vi "Configure Std Waveform.vi"(8 "error in":errorcluster, 11 "PXI-5441 Base CFG in":refnum<class "Fgen PXI CFG.lvclass">) -> (0 "error out":errorcluster, 3 "PXI-5441 Base CFG out":refnum<class "Fgen PXI CFG.lvclass">)   [LabVIEW 2023, in "HAL.lvlib" / "Fgen PXI.lvlib" / "Fgen PXI CFG.lvclass"]
uses:
  Fgen PXI CFG.lvclass
  Fgen PXI CFG.lvclass/Fgen PXI CFG.ctl
  fa98a2d5-c00a-4cbb-8575-3b170b0d9527.vi
  40d9fa99-6e9d-4d4b-a497-ff6c6c91f011.vi
  39bc53b2-902a-46e0-870e-d1b180cb98a6.vi
  c84aae48-2aac-49bb-a882-aaa71fe0ff4d.vi
  88318bc4-6f44-423c-ba11-5ee261214349.vi
  f3b2cb75-d808-412b-ab71-56c7bac84bdb.vi
  <vilib>/Utility/error.llb/Error Cluster From Error Code.vi
  <vilib>/ErrorRing/Error Ring.xnode
  4b2b93ff-10dc-4bd6-99e3-792703dd87f6.vi
  8e81885c-b6e8-4d7e-a9af-adfcbd4d7785.vi
  66779a04-485d-425c-828e-f39c11026279.vi
  Configuration Base/Configuration Base.lvclass
  fa7ec643-692d-4ae6-94d1-5cd9ea2710ab.vi
  <instrlib>/niFgen/niFgen.llb/niFgen Waveform Type.ctl
  <instrlib>/niFgen/niFgen.llb/niFgen Trigger Mode.ctl
  <instrlib>/niFgen/niFgen.llb/niFgen Output Mode.ctl
  D:/git/HAL/Configuration Base/Configuration Base.lvclass
  D:/git/HAL/Interfaces/IConfigure/IConfigure.lvclass
  D:/git/HAL/Fgen PXI/Fgen PXI CFG/Fgen PXI CFG.lvclass
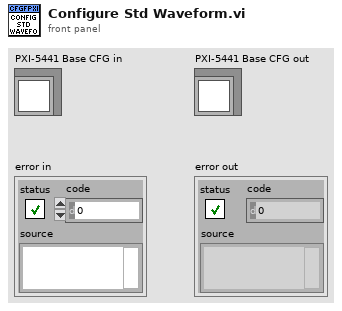
[diagram p1: front panel]
types:
  T1 = typedef "niFgen Trigger Mode.ctl" = i32
  T2 = typedef "niFgen Waveform Type.ctl" = i32
  T3 = typedef "niFgen Output Mode.ctl" = u32
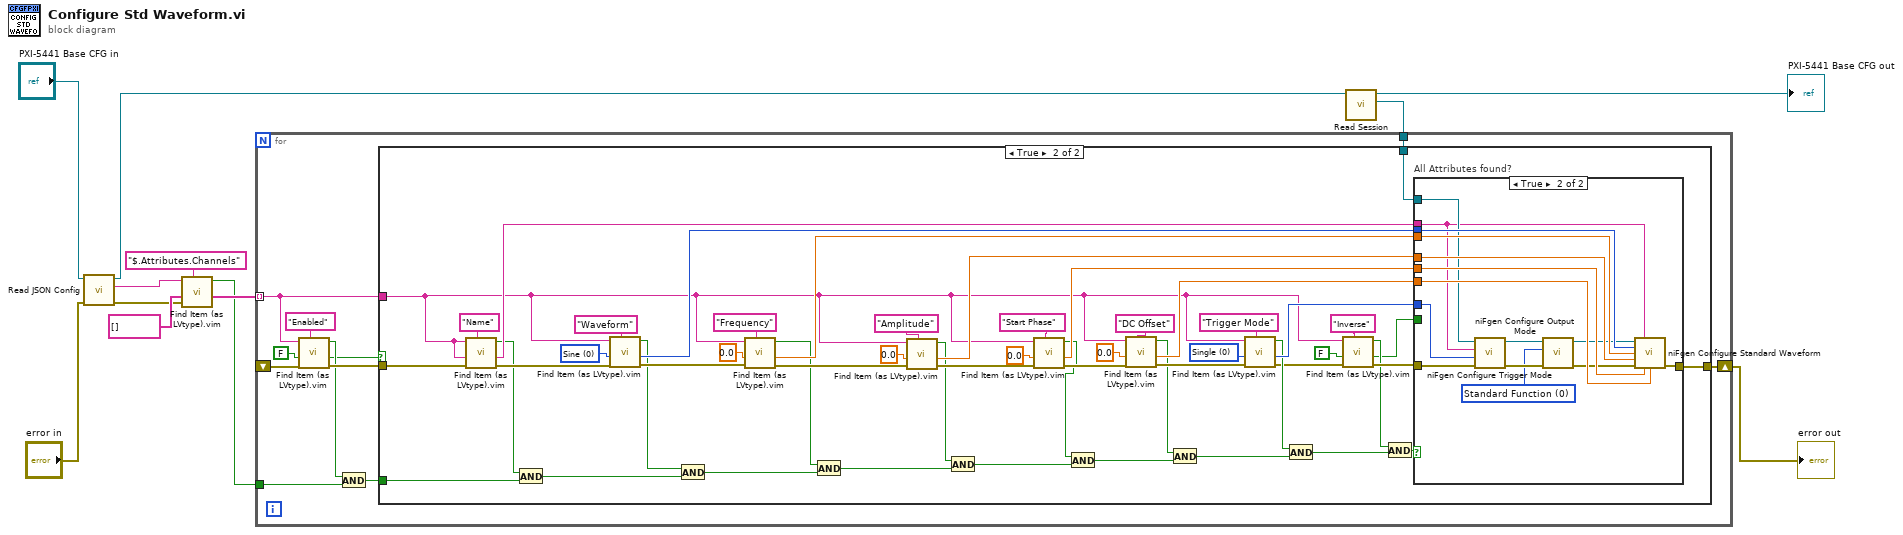
[diagram p0: block diagram]
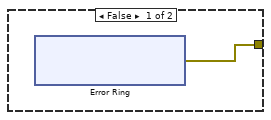
[diagram p3: hidden frame]
diagram:
  n1 = call "Read JSON Config.vi"("error in"="error in", "object in"="PXI-5441 Base CFG in") -> ("error out"=w7:errorcluster, "<JSON>Config"=w8:string, "object out"=w6:refnum<class "Fgen PXI CFG.lvclass">)  [unwired: 7 in]
  n2 = call "Find Item (as LVtype).vim"("$Path or Item Name"="$.Attributes.Channels", "error in (no error)"=w7, "Data Type and Default Value"=string[] [], "JSON"=w8) -> ("Data"=w5:string[], "Found"=w1:bool)  [unwired: 4 in, 2 out]
  n3 = call "Read Session.vi"("Fgen PXI CFG in"=w6) -> ("Session"=w4:refnum<k15>, "Fgen PXI CFG out"=→"PXI-5441 Base CFG out":refnum<class "Fgen PXI CFG.lvclass">)  [unwired: 8 in, 1 out]
  n4 = for {
    shift-right: [w23] -> w2
    shift-left: _ -> [w22]
    tunnel: w5 -> [w15] mode=indexing
    tunnel: w4 -> [w14]
    tunnel: w1 -> [w13]
    n5 = call "Find Item (as LVtype).vim"("$Path or Item Name"="Enabled", "error in (no error)"=w22, "Data Type and Default Value"=FALSE, "JSON"=w15) -> ("error out"=w21:errorcluster, "Data"=w16:bool, "Found"=w18:bool)  [unwired: 4 in, 1 out]
    n6 = And(x=w18, y=w13) -> (x .and. y?=w19:bool)
    n7 = case shown="True" w16 {
      tunnel: [w24 w76] -> w23
      tunnel: w21 -> [w24 w52]
      tunnel: w19 -> [_ w51]
      tunnel: w15 -> [_ w29]
      tunnel: w14 -> [_ w28]
      frame False {
      }
      frame True {
        w25 = T1 0 items=["Single", "Continuous", "Stepped", "Burst"] ("Trigger Mode (default: 1=continuous)")
        w27 = T2 0 items=["Sine", "Square", "Triangle", "Ramp Up", "Ramp Down", "DC", "Noise", "User"] ("Waveform")
        n8 = call "Find Item (as LVtype).vim"("$Path or Item Name"="Name", "error in (no error)"=w52, "Data Type and Default Value"=w29, "JSON"=w29) -> ("error out"=w74:errorcluster, "Data"=w64:string, "Found"=w50:bool)  [unwired: 4 in, 1 out]
        n9 = And(x=w50, y=w51) -> (x .and. y?=w48:bool)
        n10 = call "Find Item (as LVtype).vim"("$Path or Item Name"="Waveform", "error in (no error)"=w74, "Data Type and Default Value"=w27, "JSON"=w29) -> ("error out"=w73:errorcluster, "Data"=w63:T2, "Found"=w49:bool)  [unwired: 4 in, 1 out]
        n11 = And(x=w49, y=w48) -> (x .and. y?=w46:bool)
        n12 = call "Find Item (as LVtype).vim"("$Path or Item Name"="Frequency", "error in (no error)"=w73, "Data Type and Default Value"=0.0, "JSON"=w29) -> ("error out"=w69:errorcluster, "Data"=w62:dbl, "Found"=w47:bool)  [unwired: 4 in, 1 out]
        n13 = And(x=w47, y=w46) -> (x .and. y?=w44:bool)
        n14 = call "Find Item (as LVtype).vim"("$Path or Item Name"="Amplitude", "error in (no error)"=w69, "Data Type and Default Value"=0.0, "JSON"=w29) -> ("error out"=w65:errorcluster, "Data"=w61:dbl, "Found"=w45:bool)  [unwired: 4 in, 1 out]
        n15 = And(x=w45, y=w44) -> (x .and. y?=w42:bool)
        n16 = call "Find Item (as LVtype).vim"("$Path or Item Name"="Start Phase", "error in (no error)"=w65, "Data Type and Default Value"=0.0, "JSON"=w29) -> ("error out"=w58:errorcluster, "Data"=w60:dbl, "Found"=w43:bool)  [unwired: 4 in, 1 out]
        n17 = And(x=w43, y=w42) -> (x .and. y?=w40:bool)
        n18 = call "Find Item (as LVtype).vim"("$Path or Item Name"="DC Offset", "error in (no error)"=w58, "Data Type and Default Value"=0.0, "JSON"=w29) -> ("error out"=w57:errorcluster, "Data"=w56:dbl, "Found"=w41:bool)  [unwired: 4 in, 1 out]
        n19 = And(x=w41, y=w40) -> (x .and. y?=w38:bool)
        n20 = call "Find Item (as LVtype).vim"("$Path or Item Name"="Trigger Mode", "error in (no error)"=w57, "Data Type and Default Value"=w25, "JSON"=w29) -> ("error out"=w35:errorcluster, "Data"=w53:T1, "Found"=w39:bool)  [unwired: 4 in, 1 out]
        n21 = And(x=w39, y=w38) -> (x .and. y?=w37:bool)
        n22 = call "Find Item (as LVtype).vim"("$Path or Item Name"="Inverse", "error in (no error)"=w35, "Data Type and Default Value"=FALSE, "JSON"=w29) -> ("error out"=w32:errorcluster, "Data"=w30:bool, "Found"=w31:bool)  [unwired: 4 in, 1 out]
        n23 = And(x=w31, y=w37) -> (x .and. y?=w33:bool)
        n24 = case "All Attributes found?" shown="True" w33 {
          tunnel: w64 -> [_ w88]
          tunnel: w63 -> [_ w97]
          tunnel: w62 -> [_ w96]
          tunnel: w32 -> [_ w92]
          tunnel: w61 -> [_ w95]
          tunnel: w60 -> [_ w94]
          tunnel: [w77 w91] -> w76
          tunnel: w56 -> [_ w93]
          tunnel: w53 -> [_ w87]
          tunnel: w30 -> [_ _]
          tunnel: w28 -> [_ w89]
          frame False {
            n25 = xnode "Error Ring"() -> ("error out"=w77:errorcluster)
          }
          frame True {
            w83 = T3 0 items=["Standard Function", "Frequency List", "Arbitrary Waveform", "Arbitrary Sequence", "Script"] ("Output Mode (default: 0=Standard Function)")
            n26 = call <instrlib>:"niFgen Configure Trigger Mode.vi"("error in (no error)"=w92, "Trigger Mode (default: 1=continuous)"=w87, "Channel Name"=w88, "Instrument Handle"=w89) -> ("error out"=w90:errorcluster, "Instrument Handle Out"=w85:refnum<k15>)  [unwired: 6 in]
            n27 = call <instrlib>:"niFgen Configure Output Mode.vi"("error in (no error)"=w90, "Output Mode (default: 0=Standard Function)"=w83, "Instrument Handle"=w85) -> ("error out"=w86:errorcluster, "Instrument Handle Out"=w84:refnum<k15>)  [unwired: 6 in]
            n28 = call <instrlib>:"niFgen Configure Standard Waveform.vi"("Instrument Handle"=w84, "Channel Name"=w88, "Waveform"=w97, "Frequency"=w96, "Amplitude"=w95, "error in (no error)"=w86, "Start Phase"=w94, "DC Offset"=w93) -> ("error out"=w91:errorcluster)  [unwired: 6 in, 1 out]
          }
        }
      }
    }
  }
  "error out" <- w2
